vi "E05_FiltroPromediador.vi"() -> ()   [LabVIEW 2026]
panel:
  out "x/y":dbl
  in  "stop":bool
  out "Waveform Chart 2":dbl(graph)
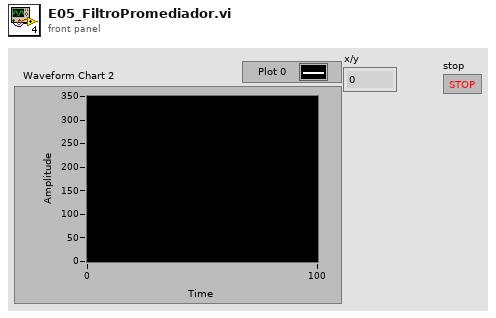
[diagram p1: front panel]
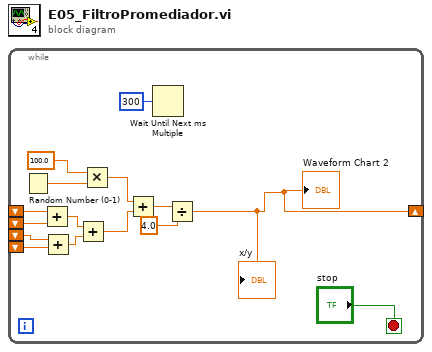
[diagram p0: block diagram]
diagram:
  n1 = while {
    shift-right: [w2] -> _
    shift-left: _ -> [w13]
    shift-left: _ -> [w10]
    shift-left: _ -> [w12]
    shift-left: _ -> [w11]
    stop <- "stop" stop-if-true
    n2 = Random Number (0-1)() -> (number: 0 to 1=w15:dbl)
    n3 = Add(x=w13, y=w12) -> (x+y=w8:dbl)
    n4 = Add(x=w11, y=w10) -> (x+y=w9:dbl)
    n5 = Add(x=w8, y=w9) -> (x+y=w7:dbl)
    n6 = Multiply(x=100.0, y=w15) -> (x*y=w6:dbl)
    n7 = Add(x=w6, y=w7) -> (x+y=w5:dbl)
    n8 = Wait Until Next ms Multiple(millisecond multiple=u32 300) -> ()  [unwired: 1 out]
    n9 = Divide(x=w5, y=4.0) -> (x/y=w2:dbl)
    "Waveform Chart 2" <- w2
    "x/y" <- w2
  }
